vi "Get Initial Standard Variation.vi"(8 "Error in":errorcluster, 11 "Beam Profiler in":refnum<class "Beam Profiler.lvclass">) -> (0 "Error out":errorcluster, 2 "Standard Variation":sgl, 3 "Beam Profiler out":refnum<class "Beam Profiler.lvclass">)   [LabVIEW 2018]
uses:
  <instrlib>/nLight Instruments/Beam Profiler/Beam Profiler.lvclass
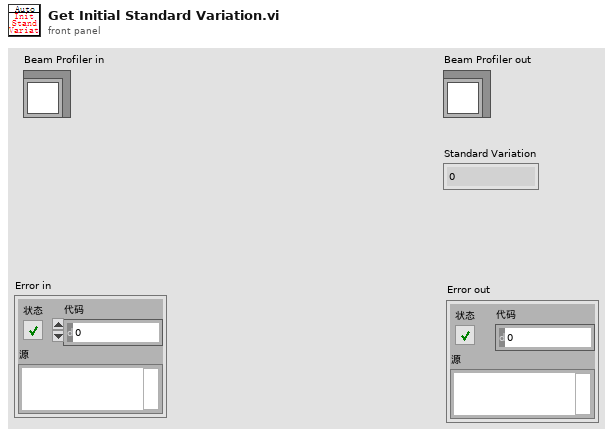
[diagram p1: front panel]
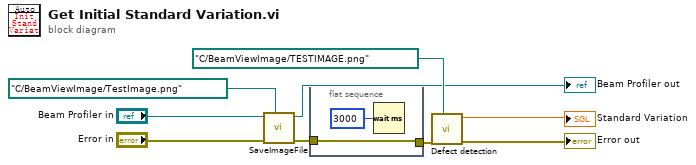
[diagram p0: block diagram]
diagram:
  n1 = call-dynamic "SaveImageFile.vi"("Path"=path "C:/BeamViewImage/TestImage.png", "error in (no error)"="Error in", "Beam Profiler in"="Beam Profiler in") -> ("error out"=w2:errorcluster, "Beam Profiler out"=→"Beam Profiler out":refnum<class "Beam Profiler.lvclass">)  [unwired: 7 in]
  n2 = flat-sequence {
    tunnel: w2 -> [w11]
    tunnel: [w11] -> w1
    frame #0 {
      n3 = Wait (ms)(milliseconds to wait=u32 3000 ("等待时间（毫秒）")) -> ()  [unwired: 1 out]
    }
  }
  n4 = call "Defect detection.vi"("File Path"=path "C:/BeamViewImage/TESTIMAGE.png", "error in"=w1) -> ("error out"=→"Error out":errorcluster, "Standard Variation"=→"Standard Variation":sgl)  [unwired: 8 in]
